vi "compare_labview_and_opengl.vi"() -> ()   [LabVIEW 2010]
uses:
  red_tweezers_paper_with_tracking/subvis/spot.ctl
  red_tweezers_paper_with_tracking/subvis/line_trapping.ctl
panel:
  out "Frame Rate":dbl
  in  "stop":bool
  in  "Spots":T1[](array[typedef])=[{"Position"={"x"=6.0125e-05, "y"=5.4187499999999996e-05, "z"=7.0069138e-06}, "Intensity"=1.0, "Vortex Charge"=0, "Phase"=1.0, "NA Position"={"x"=0.0, "y"=0.0, "r"=1.0}, "Line Trapping"={"Vector"={"x"=0.0, "y"=0.0, "z"=0.0}, "Phase Gradient"=0.0}, "Amplitude Correction"=0.0}, {"Position"={"x"=5.4116381799999997e-05, "y"=3.98060334e-05, "z"=0.0}, "Intensity"=1.0, "Vortex Charge"=0, "Phase"=1.0, "NA Position"={"x"=0.0, "y"=0.0, "r"=1.0}, "Line Trapping"={"Vector"={"x"=0.0, "y"=0.0, "z"=0.0}, "Phase Gradient"=0.0}, "Amplitude Correction"=0.0}, {"Position"={"x"=7.662499999999999e-05, "y"=4.6e-05, "z"=0.0}, "Intensity"=1.0, "Vortex Charge"=0, "Phase"=1.0, "NA Position"={"x"=0.0, "y"=0.0, "r"=1.0}, "Line Trapping"={"Vector"={"x"=0.0, "y"=0.0, "z"=0.0}, "Phase Gradient"=0.0}, "Amplitude Correction"=0.0}] {"Amplitude Correction" step=0.1; "Line Trapping"."Phase Gradient" step=0.05; "Line Trapping"."Vector"."x" step=1e-06 format="%#_6p"; "Line Trapping"."Vector"."y" step=1e-06 format="%#_6p"; "Line Trapping"."Vector"."z" step=1e-06 format="%#_6p"; "NA Position"."r" step=1e-06; "NA Position"."y" step=1e-06; "NA Position"."x" step=1e-06; "Position"."z" step=1e-06; "Position"."y" step=1e-06; "Position"."x" step=1e-06; "Phase" step=0.7753; "Intensity" step=0.1}
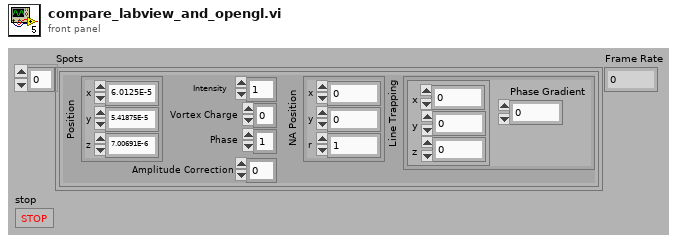
[diagram p1: front panel]
types:
  T1 = typedef "spot.ctl" = cluster{"Position":cluster{"x":dbl, "y":dbl, "z":dbl}, "Intensity":dbl, "Vortex Charge":i8, "Phase":dbl, "NA Position":cluster{"x":dbl, "y":dbl, "r":dbl}, "Line Trapping":T2, "Amplitude Correction":dbl}
  T2 = typedef "line_trapping.ctl" = cluster{"Vector":cluster{"x":dbl, "y":dbl, "z":dbl}, "Phase Gradient":dbl}
  T3 = cluster{"Average Frame Time":dbl, "millisecond timer value":u32}
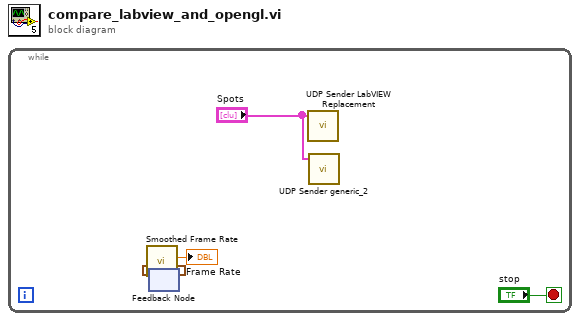
[diagram p0: block diagram]
diagram:
  n1 = while {
    stop <- "stop" stop-if-true
    n2 = feedback #1() -> (w1:T3)  [unwired: 1 in]
    n3 = call "Smoothed Frame Rate.vi"("Feedback In"=w1) -> ("Feedback Out"=w2:T3, "Frame Rate"=→"Frame Rate":dbl)  [unwired: 5 in]
    n4 = feedback-in #1(w2) -> ()
    n5 = call "UDP Sender LabVIEW Replacement.vi"("Spots"="Spots") -> ()  [unwired: 3 in]
    n6 = call "UDP Sender generic_2.vi"("Spots"="Spots") -> ()  [unwired: 2 in, 1 out]
  }
